vi "Wrist.vi"(0 "WristInput":dbl, 1 "WristSetpoint":dbl, 2 "WristSweet":bool) -> ()   [LabVIEW 2017]
uses:
  Phoenix-LabVIEW/Motor Controller/Controls/CTRE_Phoenix_MotorControl_ControlMode.ctl
  Robot Global Data.vi
panel:
  in  "In":dbl=-1.0 format="%#_13g"
  in  "Down":dbl=1.45 format="%#_13g"
  in  "SoftStop":dbl=-0.5 format="%#_13g"
  in  "Wrist G":dbl=-0.1 format="%#_13g"
  in  "WristMax":dbl=0.55
  in  "WristP":dbl=-0.6 format="%#_13g"
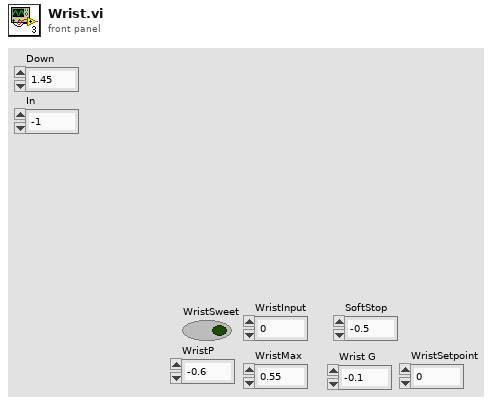
[diagram p1: front panel]
types:
  T1 = typedef "CTRE_Phoenix_MotorControl_ControlMode.ctl" = u16
  T2 = typedef "WPI_MotorControlDeviceRef.ctl" = cluster{"DeviceStatus":errorcluster, "Type":T3, "PWM":cluster{"PWM Channel":T4, "DeadBand":T5}, "CAN":cluster{"Device Number":u8, "SetOutput VI Ref":variant, "GetOutput VI Ref":variant, "Enable VI Ref":variant, "Disable VI Ref":variant, "Data":variant}, "Invert":bool, "DIO PWM":cluster{"PWM \"Enable\" Channel":T4, "DIOChannel":T6, "PWM Rate":dbl}}
  T3 = typedef "WPI_MotorControlType.ctl" = enum16{"PWM", "CAN", "DIO PWM"}
  T4 = typedef "FPGA_DIOPWMChannel.ctl" = enum8{"PWM 0", "PWM 1", "PWM 2", "PWM 3", "PWM 4", "PWM 5", "PWM 6", "PWM 7", "PWM 8", "PWM 9", "PWM MXP 0", "PWM MXP 1", "PWM MXP 2", "PWM MXP 3", "PWM MXP 4", "PWM MXP 5", "PWM MXP 6", "PWM MXP 7", "PWM MXP 8", "PWM MXP 9", "Invalid"}
  T5 = typedef "WPI_PWMDeadband.ctl" = cluster{"Name":string, "maxPositivePwm":i32, "minPositivePwm":i32, "centerPwm":i32, "maxNegativePwm":i32, "minNegativePwm":i32, "angularRange":u16}
  T6 = typedef "FPGA_DIOChannel.ctl" = enum8{"DIO 0", "DIO 1", "DIO 2", "DIO 3", "DIO 4", "DIO 5", "DIO 6", "DIO 7", "DIO 8", "DIO 9", "DIO MXP 0", "DIO MXP 1", "DIO MXP 2", "DIO MXP 3", "DIO MXP 4", "DIO MXP 5", "DIO MXP 6", "DIO MXP 7", "DIO MXP 8", "DIO MXP 9", "DIO MXP 10", "DIO MXP 11", "DIO MXP 12", "DIO MXP 13", "DIO MXP 14", "DIO MXP 15", "SPI Port CS1", "SPI Port CS2", "SPI Port CS3", "SPI Port MISO", "SPI Port MOSI", "Invalid"}
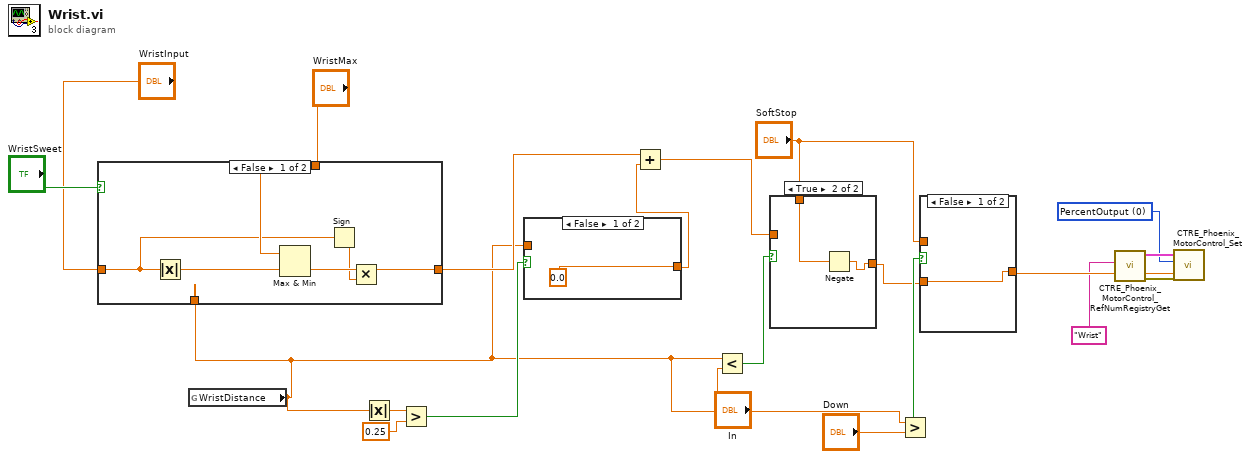
[diagram p0: block diagram]
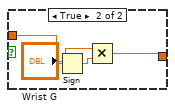
[diagram p4: hidden frame]
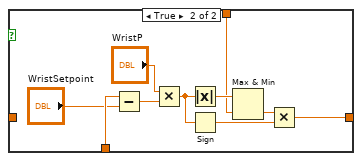
[diagram p5: hidden frame]
diagram:
  w1 = T1 0 items=["PercentOutput"=0, "Position"=1, "Velocity"=2, "Current"=3, "Follower"=5, "MotionProfile"=6, "MotionMagic"=7, "MotionMagicArc"=8, "MotionProfileArc"=10, "Disabled"=15] ("Control Mode")
  n1 = global read "Robot Global Data.vi" "WristDistance"() -> (w6:dbl)
  n2 = case shown="False" "WristSweet" {
    tunnel: "WristMax" -> [w26 w33]
    tunnel: [w24 w31] -> w15
    tunnel: "WristInput" -> [w22 _]
    tunnel: w6 -> [_ w29]
    frame False {
      n3 = Absolute Value(x=w22) -> (abs(x)=w25:dbl)
      n4 = Max & Min(x=w26, y=w25) -> (min(x,y)=w27:dbl)  [unwired: 1 out]
      n5 = Sign(1:w22) -> (0:w23:dbl)
      n6 = Multiply(x=w27, y=w23) -> (x*y=w24:dbl)
    }
    frame True {
      n7 = Subtract(x=w29, y="WristSetpoint") -> (x-y=w30:dbl)
      n8 = Multiply(x="WristP", y=w30) -> (x*y=w32:dbl)
      n9 = Absolute Value(x=w32) -> (abs(x)=w34:dbl)
      n10 = Sign(1:w32) -> (0:w35:dbl)
      n11 = Max & Min(x=w34, y=w33) -> (min(x,y)=w36:dbl)  [unwired: 1 out]
      n12 = Multiply(x=w36, y=w35) -> (x*y=w31:dbl)
    }
  }
  n13 = Absolute Value(x=w6) -> (abs(x)=w18:dbl)
  n14 = Greater?(x=w18, y=0.25) -> (0:w16:bool)
  n15 = case shown="False" w16 {
    tunnel: [0.0 w40] -> w14
    tunnel: w6 -> [_ w41]
    frame False {
    }
    frame True {
      n16 = Sign(1:w41) -> (0:w42:dbl)
      n17 = Multiply(x="Wrist G", y=w42) -> (x*y=w40:dbl)
    }
  }
  n18 = Add(x=w15, y=w14) -> (x+y=w5:dbl)
  n19 = Less?(x=w6, y="In") -> (x < y?=w12:bool)
  n20 = case shown="True" w12 {
    tunnel: [w43 w45] -> w7
    tunnel: "SoftStop" -> [_ w44]
    tunnel: w5 -> [w43 _]
    frame False {
    }
    frame True {
      n21 = Negate(x=w44) -> (-x=w45:dbl)
    }
  }
  n22 = Greater?(x=w6, y="Down") -> (0:w10:bool)
  n23 = case shown="False" w10 {
    tunnel: [w46 w47] -> w9
    tunnel: "SoftStop" -> [_ w47]
    tunnel: w7 -> [w46 _]
    frame False {
    }
    frame True {
    }
  }
  n24 = call "CTRE_Phoenix_MotorControl_RefNumRegistryGet.vi"("refnum name"="Wrist") -> ("error out"=w3:errorcluster, "PhoenixMotorControlDevRef"=w4:T2)  [unwired: 9 in]
  n25 = call "CTRE_Phoenix_MotorControl_Set.vi"("error in (no error)"=w3, "Output"=w9, "Control Mode"=w1, "PhoenixMotorControlDevRef"=w4) -> ()  [unwired: 6 in, 2 out]
